vi "mod_FractionalResampler.vi"(0 "samples in":cdb[](array[numeric]), 5 "resampler state in":T1, 7 "offset":dbl, 9 "rate factor":dbl, 11 "error in (no error)":errorcluster, 12 "reset":bool=TRUE, 13 "flush":bool) -> (4 "samples out":cdb[](array[numeric]), 6 "resampler state out":T1, 15 "error out":errorcluster)   [LabVIEW 2020, in "niAMT.lvlib"]
uses:
  <vilib>/addons/Modulation/niAMT.lvlib
  <vilib>/addons/Modulation/Analog/controls/mod_ResamplerState.ctl
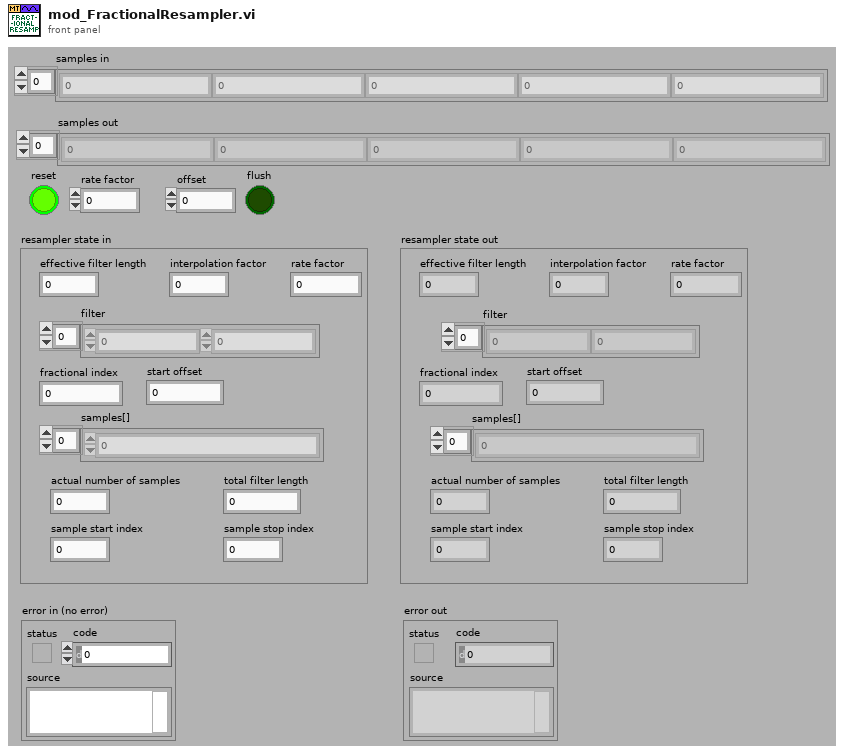
[diagram p1: front panel]
types:
  T1 = typedef "niAMT.lvlib/mod_ResamplerState.ctl" = cluster{"effective filter length":i32, "interpolation factor":i32, "rate factor":dbl, "filter":dbl[], "fractional index":dbl, "start offset":i32, "samples[]":cdb[], "actual number of samples":i32, "total filter length":i32, "sample start index":i32, "sample stop index":i32}
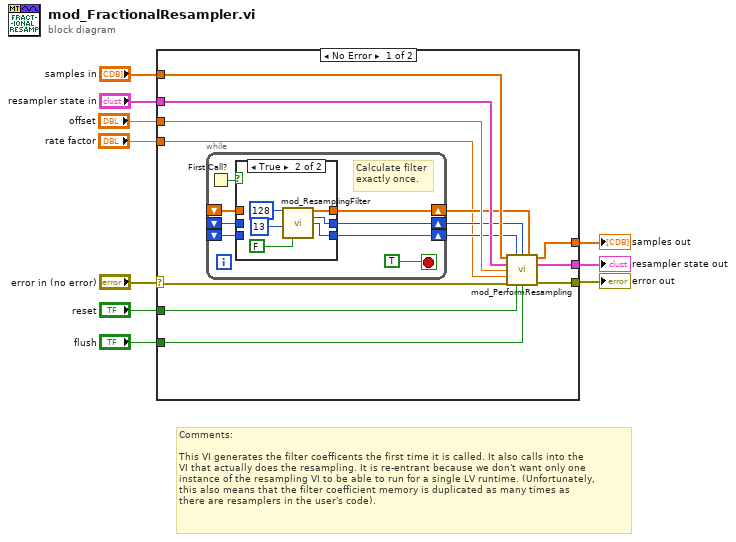
[diagram p0: block diagram]
diagram:
  # "Comments:\n\nThis VI generates the filter coefficents the first time it is called. It also calls into the\nVI that actually does the resampling. It is re-entrant because we don't want only one\ninstance of the resampling VI to be able to run for a single LV runtime. (Unfortunately,\nthis also means that the filter coefficient memory is duplicated as many times as \nthere are resamplers in the user's code)."
  n1 = case shown="No Error" "error in (no error)" {
    selector: "error in (no error)" -> [w13 w41]
    tunnel: "samples in" -> [w22 w43]
    tunnel: "resampler state in" -> [w21 w42]
    tunnel: [w20 w42] -> w8
    tunnel: "offset" -> [w17 _]
    tunnel: "reset" -> [w18 _]
    tunnel: [w19 w43] -> w5
    tunnel: [w23 w41] -> w3
    tunnel: "rate factor" -> [w11 _]
    tunnel: "flush" -> [w12 _]
    frame No Error {
      n2 = while {
        shift-right: [w31] -> w16
        shift-left: _ -> [w26]
        shift-right: [w30] -> w15
        shift-left: _ -> [w27]
        shift-right: [w29] -> w14
        shift-left: _ -> [w28]
        stop <- TRUE stop-if-true
        # "Calculate filter\nexactly once."
        n3 = First Call?() -> (First Call?: T/F=w25:bool)
        n4 = case shown="True" w25 {
          tunnel: [w32 w38] -> w31
          tunnel: [w33 w37] -> w30
          tunnel: [w34 w36] -> w29
          tunnel: w28 -> [w34 _]
          tunnel: w27 -> [w33 _]
          tunnel: w26 -> [w32 _]
          frame False {
          }
          frame True {
            n5 = call <vilib>:"mod_ResamplingFilter.vi"("interpolation factor in"=128, "effective filter length"=13, "legacy filter?"=FALSE) -> ("filerData[]"=w38:dbl[], "interpolation factor"=w37:i32, "effective filter length"=w36:i32)  [unwired: 1 in, 9 out]
          }
        }
      }
      n6 = call <vilib>:"mod_PerformResampling.vi"("samples in"=w22, "effective filter length"=w14, "interpolation factor"=w15, "filterData"=w16, "resampler state in"=w21, "offset"=w17, "rate factor"=w11, "error in (no error)"=w13, "reset"=w18, "flush"=w12) -> ("samples out"=w19:cdb[], "resampler state out"=w20:T1, "error out"=w23:errorcluster)  [unwired: 3 out]
    }
    frame Error {
    }
  }
  "samples out" <- w5
  "resampler state out" <- w8
  "error out" <- w3
